vi "get freq byte.vi"(8 "error in (no error)":errorcluster caption="에러 입력(에러 없음)", 10 "freq":u32, 11 "Haptic IC 입력":refnum<class "Haptic IC.lvclass">) -> (0 "error out":errorcluster caption="에러 출력", 2 "byte value":u8 format="%02x", 3 "Haptic IC 출력":refnum<class "Haptic IC.lvclass">)   [LabVIEW 2020, in "Haptic IC.lvclass"]
uses:
  Haptic IC.lvclass
  d21bd180-1394-4622-81d1-d93d71beaaf2.vi
  <vilib>/Comparison/Equal/Equal Functor/Equal Functor.lvclass
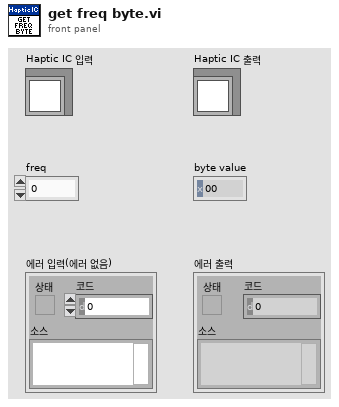
[diagram p1: front panel]
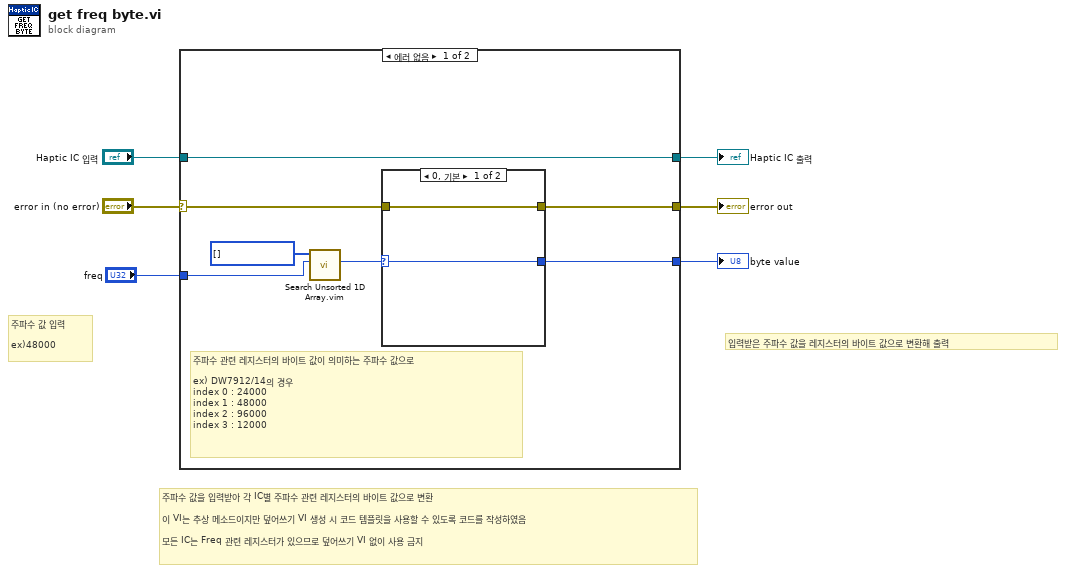
[diagram p0: block diagram]
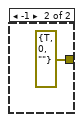
[diagram p2: hidden frame]
diagram:
  # "입력받은 주파수 값을 레지스터의 바이트 값으로 변환해 출력"
  # "주파수 값 입력\n\nex)48000"
  # "주파수 값을 입력받아 각 IC별 주파수 관련 레지스터의 바이트 값으로 변환\n\n이 VI는 추상 메소드이지만 덮어쓰기 VI 생성 시 코드 템플릿을 사용할 수 있도록 코드를 작성하였음\n\n모든 IC는 Freq 관련 레지스터가 있으므로 덮어쓰기 VI 없이 사용 금지"
  n1 = case shown="에러 없음" "error in (no error)" {
    selector: "error in (no error)" -> [w10 w18]
    tunnel: [w7 w18] -> w3
    tunnel: "Haptic IC 입력" -> [w13 w17]
    tunnel: [w13 w17] -> w5
    tunnel: "freq" -> [w11 _]
    tunnel: [w8 _] -> w1
    frame No Error {
      # "주파수 관련 레지스터의 바이트 값이 의미하는 주파수 값으로\n\nex) DW7912/14의 경우\nindex 0 : 24000\nindex 1 : 48000\nindex 2 : 96000\nindex 3 : 12000"
      n2 = call "Search Unsorted 1D Array.vim"("element"=w11, "unsorted 1D array"=u32[] []) -> ("index of element"=w9:i32)  [unwired: 9 in]
      n3 = case shown="0, 기본" w9 {
        selector: w9 -> [w15 _]
        tunnel: w10 -> [w14 _]
        tunnel: [w15 _] -> w8
        tunnel: [w14 errorcluster {"status"=TRUE, "code"=0, "source"=""} ("error IO")] -> w7
        frame 0, Default {
        }
        frame -1 {
        }
      }
    }
    frame Error {
    }
  }
  "error out" <- w3
  "Haptic IC 출력" <- w5
  "byte value" <- w1
